vi "XIPIN_MicroBlaze_MCS_1_4.vi"   [LabVIEW 2017]
doc: "MicroBlaze Micro Controller System (MCS) is a light-weight general purpose micro controller system, based on the MicroBlaze processor. It is primarily intended for simple control applications, where a hardware solution would be less flexible and more difficult to implement. Software development with the Xilinx Software Development Kit (SDK) is supported, including a software driver for the peripherals. Debugging is available either via SDK or directly with the Xilinx Microprocessor Debugger.\n\nThe MCS consists of the processor itself, local memory with sizes ranging from 4KB to 64KB, up to 4 Fixed Interval Timers, up to 4 Programmable Interval Timers, up to 4 32-bit General Purpose Output ports, up to 4 32-bit General Purpose Input ports, and an Interrupt Controller with up to 16 external interrupt inputs.\n\n------------------------------------\n<b>Need License</b> : No"
uses:
  <vilib>/rvi/XilinxIP/XIPIN_XNode/niFpgaXIPIN.xnode
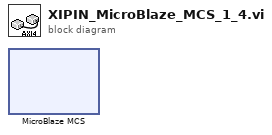
[diagram p0: block diagram]
diagram:
  n1 = xnode ("MicroBlaze MCS")() -> ()
